vi "JSON title read.vi"(8 "error in (no error)":errorcluster, 10 "<JSON> in":string[](array[string]), 11 "Item Names":string[](array[string])) -> (0 "error out":errorcluster, 3 "<JSON> out":string)   [LabVIEW 2019]
uses:
  <vilib>/Utility/error.llb/Error Cluster From Error Code.vi
  <vilib>/ErrorRing/Error Ring.xnode
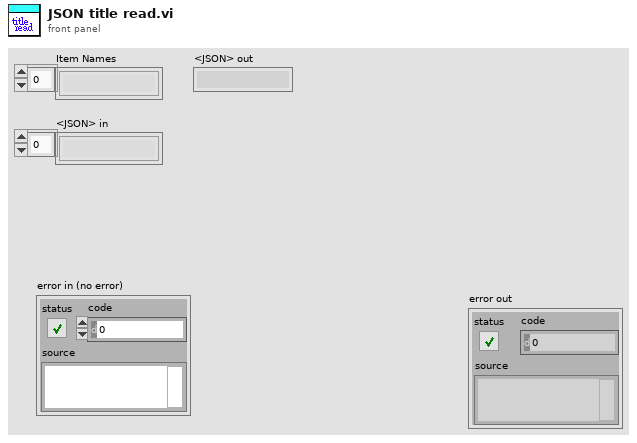
[diagram p1: front panel]
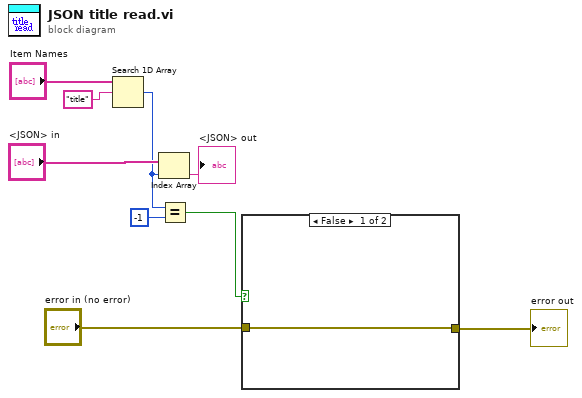
[diagram p0: block diagram]
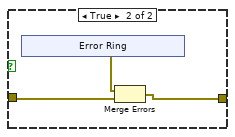
[diagram p2: hidden frame]
diagram:
  n1 = Search 1D Array(1D array="Item Names", element="title") -> (index of element=w5:i32)  [unwired: 1 in]
  n2 = Index Array(array="<JSON> in", index=w5) -> (element=→"<JSON> out":string)
  n3 = Equal?(x=w5, y=-1) -> (x = y?=w3:bool)
  n4 = case shown="False" w3 {
    tunnel: "error in (no error)" -> [w10 w13]
    tunnel: [w10 w11] -> w1
    frame False {
    }
    frame True {
      n5 = xnode "Error Ring"() -> ("error out"=w12:errorcluster)
      n6 = Merge Errors(w12, w13) -> (w11:errorcluster)
    }
  }
  "error out" <- w1
